vi "setParameters.vi"(10 "Parameters":T1, 11 "ShutdownCommand in":refnum<class "ShutdownCommand.lvclass">) -> (3 "ShutdownCommand out":refnum<class "ShutdownCommand.lvclass">)   [LabVIEW 2016, in "ShutdownCommand.lvclass"]
uses:
  ShutdownCommand.lvclass
  DataTypes/Topics/CommandShutdown.ctl
  DataTypes/Topics/Parts/CommandId.ctl
  ShutdownCommand.lvclass/ShutdownCommand.ctl
  DataTypes/Topics/M1M3SupportTopics.lvlib
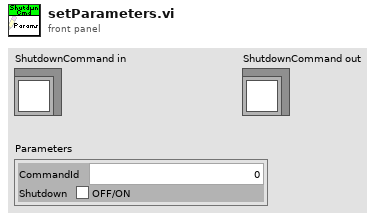
[diagram p1: front panel]
types:
  T1 = typedef "M1M3SupportTopics.lvlib/CommandShutdown.ctl" = cluster{"CommandId":T2, "Shutdown":bool}
  T2 = typedef "M1M3SupportTopics.lvlib/CommandId.ctl" = i32
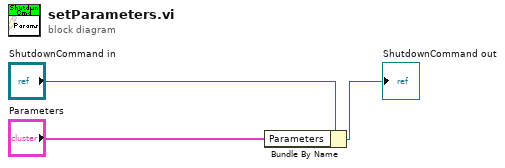
[diagram p0: block diagram]
diagram:
  n1 = Bundle By Name(cluster="ShutdownCommand in", "Parameters"="Parameters") -> (→"ShutdownCommand out":refnum<class "ShutdownCommand.lvclass">)
